vi "PXI-Config DAQmx AI.vi"(0 "task in":refnum<k21>, 11 "error in":errorcluster) -> (4 "task out":refnum<k21>, 15 "error out":errorcluster)   [LabVIEW 2020]
uses:
  <resource>/objmgr/daqmx.rc
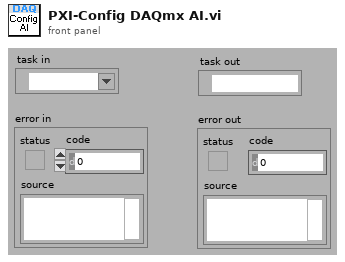
[diagram p1: front panel]
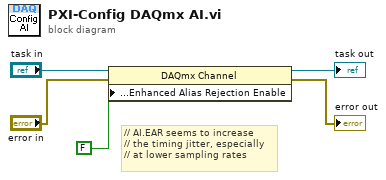
[diagram p0: block diagram]
diagram:
  # "// AI.EAR seems to increase\n// the timing jitter, especially\n// at lower sampling rates"
  n1 = property class="DAQmx Channel"(reference="task in", error in="error in", "Analog Input:General Properties:Advanced:Enhanced Alias Rejection Enable"=FALSE) -> (reference out=→"task out":refnum<k21>, error out=→"error out":errorcluster)
